vi "bin array to shotnumber array.vi"(11 "Bin Group":i32[](array[numeric])) -> (3 "Shot numbers":i32[](array[numeric]))   [LabVIEW 2020]
uses:
  <userlib>/_OpenG.lib/array/array.llb/Search 1D Array (I32)__ogtk.vi
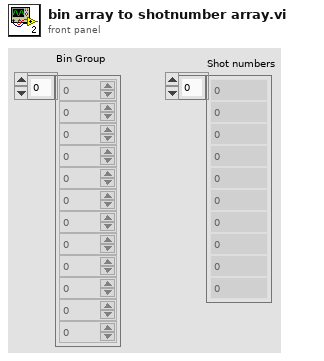
[diagram p1: front panel]
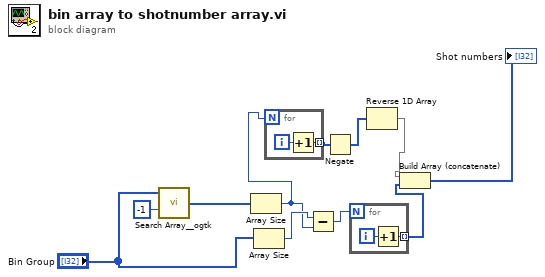
[diagram p0: block diagram]
diagram:
  n1 = call-poly <userlib>:"Search Array__ogtk.vi"("Array"="Bin Group", "Element Data"=-1 ("Bin Group")) -> ("Indices of Elements"=w6:i32[])  [unwired: 7 in]
  n2 = Array Size(array=w6) -> (size(s)=w4:i32)
  n3 = Array Size(array="Bin Group") -> (size(s)=w9:i32)
  n4 = for {
    N: w4 -> [_]
    tunnel: [w12] -> w3 mode=indexing
    i -> [w13]
    n5 = Increment(x=w13) -> (x+1=w12:i32)
  }
  n6 = Subtract(x=w9, y=w4) -> (x-y=w10:i32)
  n7 = Negate(x=w3) -> (-x=w2:i32[])
  n8 = for {
    N: w10 -> [_]
    tunnel: [w14] -> w11 mode=indexing
    i -> [w15]
    n9 = Increment(x=w15) -> (x+1=w14:i32)
  }
  n10 = Reverse 1D Array(array=w2) -> (reversed array=w1:i32[])
  n11 = Build Array (concatenate)(w1, w11) -> (→"Shot numbers":i32[])
